vi "Refresh.vi"(8 "error in (no error)":errorcluster, 10 "Engine Configuration In":refnum<class "engine configuration.lvclass">, 11 "CVT editor node In":refnum<class "CVT editor node.lvclass">) -> (0 "error out":errorcluster, 2 "Engine Configuration Out":refnum<class "engine configuration.lvclass">, 3 "CVT editor node Out":refnum<class "CVT editor node.lvclass">)   [LabVIEW 2013, in "CVT editor node.lvclass"]
uses:
  CVT editor node.lvclass
  <vilib>/NI/Module Execution Interface/Engine Configuration/engine configuration.lvclass
  configuration/CVT configuration.lvclass
  <vilib>/NI/Tag Bus Data Framework/Configuration Editor/Classes/Module editor node/Read Module Configuration.vi
  <vilib>/NI/Tag Bus Data Framework/Configuration Editor/Classes/Module editor node/Write Module Configuration.vi
  <vilib>/NI/Tag Bus Module Framework/module configuration/TBM module configuration.lvclass
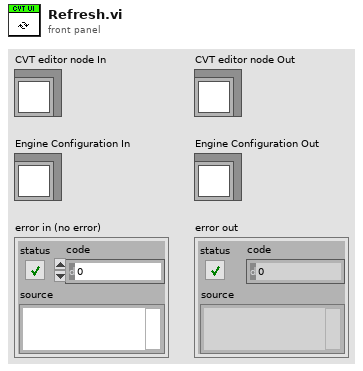
[diagram p1: front panel]
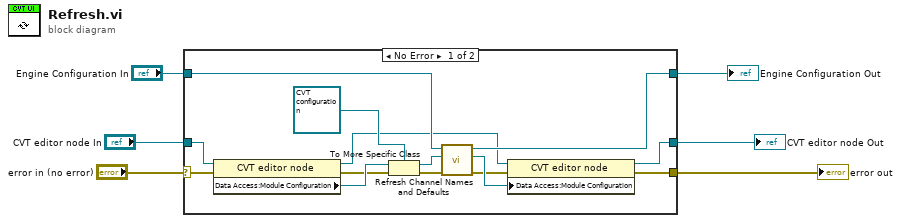
[diagram p0: block diagram]
diagram:
  n1 = case shown="No Error" "error in (no error)" {
    selector: "error in (no error)" -> [w10 w21]
    tunnel: "Engine Configuration In" -> [w20 w23]
    tunnel: "CVT editor node In" -> [w19 w22]
    tunnel: [w14 w22] -> w4
    tunnel: [w8 w21] -> w3
    tunnel: [w13 w23] -> w2
    frame No Error {
      n2 = property class="CVT editor node"(reference=w19, error in=w10) -> (reference out=w7:refnum<class "CVT editor node.lvclass">, error out=w12:errorcluster, "Data Access:Module Configuration"=w15:refnum<class "TBM module configuration.lvclass">)
      n3 = To More Specific Class(target class=refnum<class "CVT configuration.lvclass"> refnum ("CVT configuration"), reference=w15, error in=w12) -> (specific class reference=w17:refnum<class "CVT configuration.lvclass">, error out=w11:errorcluster)
      n4 = call "Refresh Channel Names and Defaults.vi"("error in (no error)"=w11, "CVT configuration in"=w17, "engine configuration in"=w20) -> ("error out"=w9:errorcluster, "CVT configuration out"=w18:refnum<class "CVT configuration.lvclass">, "engine configuration out"=w13:refnum<class "engine configuration.lvclass">)  [unwired: 6 in]
      n5 = property class="CVT editor node"(reference=w7, error in=w9, "Data Access:Module Configuration"=w18) -> (reference out=w14:refnum<class "CVT editor node.lvclass">, error out=w8:errorcluster)
    }
    frame Error {
    }
  }
  "CVT editor node Out" <- w4
  "error out" <- w3
  "Engine Configuration Out" <- w2
